vi "checkMove.vi"(8 "error in (no error)":errorcluster, 11 "Simon_Engine in":refnum<class "Simon_Engine.lvclass">) -> (0 "error out":errorcluster, 2 "MachStatus":i16, 3 "Simon_Engine out":refnum<class "Simon_Engine.lvclass">)   [LabVIEW 2019, in "Simon_Engine.lvclass"]
doc: "Check if the sequence entered by the player matches with the generated sequence. This method tests each user input individually."
uses:
  Simon_Engine.lvclass
  Simon_Engine.lvclass/Simon_Engine.ctl
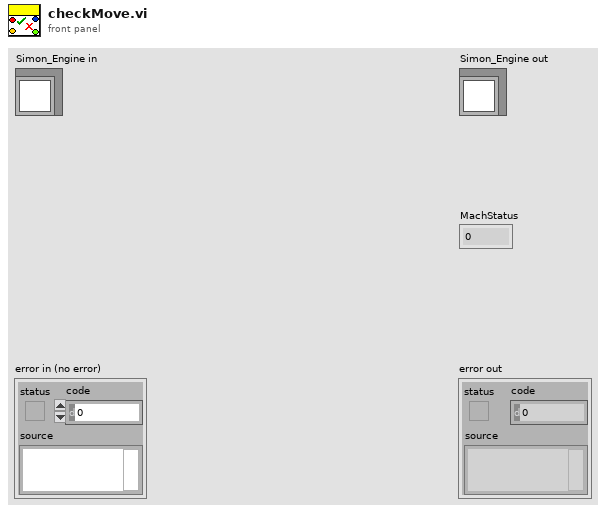
[diagram p1: front panel]
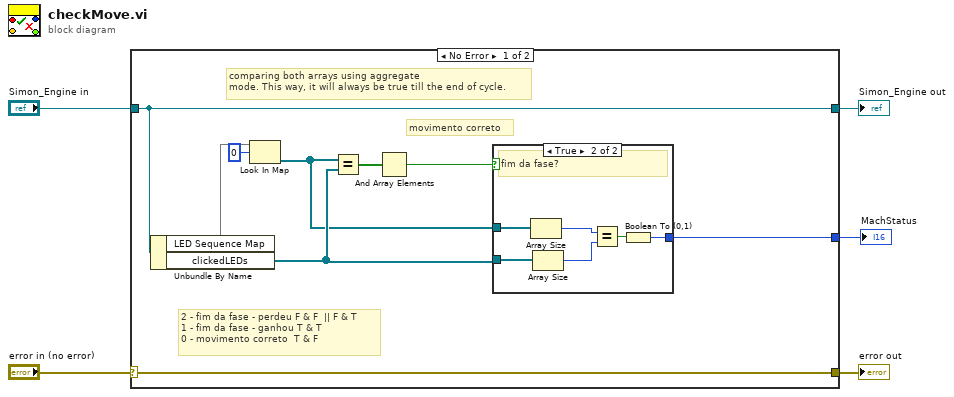
[diagram p0: block diagram]
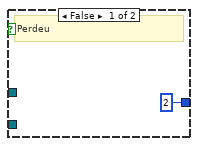
[diagram p2: hidden frame]
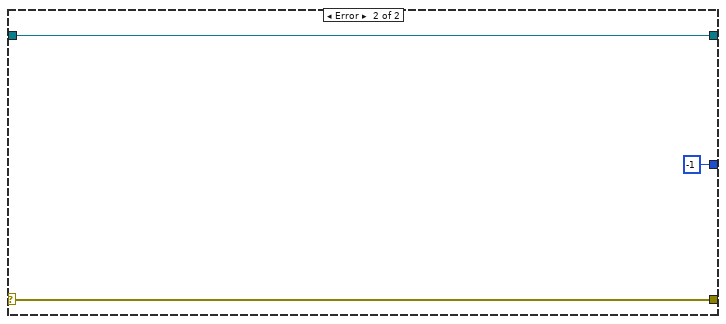
[diagram p3: hidden frame]
diagram:
  n1 = case shown="No Error" "error in (no error)" {
    selector: "error in (no error)" -> [w13 w24]
    tunnel: [w13 w24] -> w4
    tunnel: [w14 w23] -> w2
    tunnel: "Simon_Engine in" -> [w14 w23]
    tunnel: [w9 i16 -1] -> w1
    frame No Error {
      # "2 - fim da fase - perdeu F & F  || F & T\n1 - fim da fase - ganhou T & T\n0 - movimento correto  T & F"
      # "movimento correto"
      # "comparing both arrays using aggregate\nmode. This way, it will always be true till the end of cycle."
      n2 = Unbundle By Name(w14) -> ("LED Sequence Map"=w7:map{u8, refnum<class "LED.lvclass">[]}, "clickedLEDs"=w10:refnum<class "LED.lvclass">[])
      n3 = Look In Map(map=w7, key=u8 0) -> (value=w8:refnum<class "LED.lvclass">[])  [unwired: 1 in, 1 out]
      n4 = Equal?(x=w8, y=w10) -> (x = y?=w12:bool[])
      n5 = And Array Elements(Boolean array=w12) -> (logical AND=w11:bool)
      n6 = case shown="True" w11 {
        tunnel: w10 -> [_ w19]
        tunnel: w8 -> [_ w18]
        tunnel: [i16 2 w16] -> w9
        frame False {
          # "Perdeu"
        }
        frame True {
          # "fim da fase?"
          n7 = Array Size(array=w18) -> (size(s)=w20:i32)
          n8 = Array Size(array=w19) -> (size(s)=w21:i32)
          n9 = Equal?(x=w20, y=w21) -> (x = y?=w17:bool)
          n10 = Boolean To (0,1)(Boolean=w17) -> (0, 1=w16:i16)
        }
      }
    }
    frame Error {
    }
  }
  "error out" <- w4
  "Simon_Engine out" <- w2
  "MachStatus" <- w1
